vi "Create Message Queue.vi"(8 "error in (no error)":errorcluster, 9 "Initial Message Values":string[](array[string]), 10 "Initial Message Names":string[](array[string]), 11 "Message Queue Name":string) -> (0 "error out":errorcluster, 3 "Message Queue out":T1)   [LabVIEW 2014, in "AMC.lvlib"]
doc: "This VI creates a new local message queue or returns a reference to an existing message queue baseed on the queue name. You can pass in a list of initial messages which will be added to the queue."
uses:
  AMC.lvlib
  _SubVIs/TypeDefs/Message Queue.ctl
  _SubVIs/TypeDefs/Message.ctl
  Keyed Array/KeyedArray.ctl
  Keyed Array/Tools_KeyedArray.lvlib
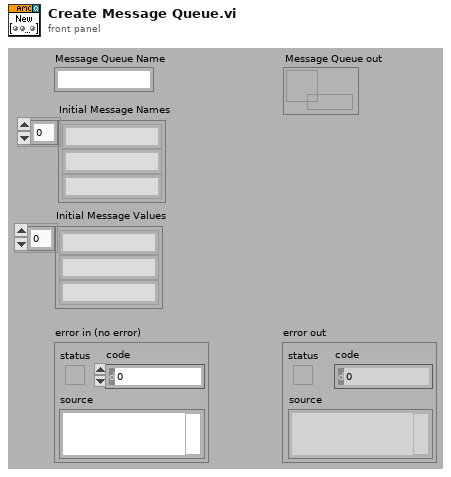
[diagram p1: front panel]
types:
  T1 = typedef "AMC.lvlib/Message Queue.ctl" = refnum<queue>
  T2 = typedef "AMC.lvlib/Message.ctl" = cluster{"Name":string, "Value":string, "Attributes":T3, "Receiver Host":string, "Receiver Process":string, "Source Host":string, "Source Process":string, "Priority Message":bool, "Acknowledge Message":bool}
  T3 = typedef "Tools_KeyedArray.lvlib/KeyedArray.ctl" = cluster{"keys":string[], "values":string[]}
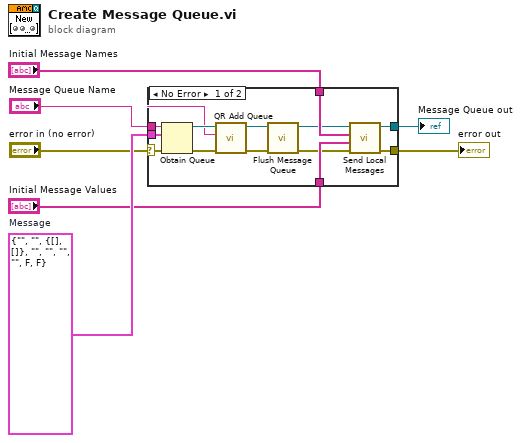
[diagram p0: block diagram]
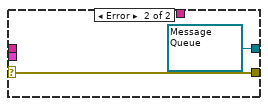
[diagram p2: hidden frame]
diagram:
  w7 = T2 {"Name"="", "Value"="", "Attributes"={"keys"=[], "values"=[]}, "Receiver Host"="", "Receiver Process"="", "Source Host"="", "Source Process"="", "Priority Message"=FALSE, "Acknowledge Message"=FALSE}  # Message
  n1 = case shown="No Error" "error in (no error)" {
    selector: "error in (no error)" -> [w8 w22]
    tunnel: w7 -> [w20 _]
    tunnel: [w19 w22] -> w6
    tunnel: [w18 T1 refnum ("Message Queue out")] -> w5
    tunnel: "Initial Message Names" -> [w17 _]
    tunnel: "Initial Message Values" -> [w16 _]
    tunnel: "Message Queue Name" -> [w13 _]
    frame No Error {
      n2 = Obtain Queue(name (unnamed)=w13, element data type=w20, error in (no error)=w8) -> (queue out=w14:refnum<queue>, error out=w15:errorcluster)  [unwired: 2 in, 1 out]
      n3 = call "QR Add Queue .vi"("error in (no error)"=w15, "Name"=w13, "Message Queue in"=w14) -> ("error out"=w12:errorcluster, "Message Queue out"=w11:T1)  [unwired: 7 out]
      n4 = call "Flush Message Queue.vi"("error in (no error)"=w12, "Message Queue in"=w11) -> ("error out"=w9:errorcluster, "Message Queue out"=w10:T1)  [unwired: 7 out]
      n5 = call "Send Local Messages.vi"("error in (no error)"=w9, "Message Values"=w16, "Message Names"=w17, "Message Queue in"=w10) -> ("error out"=w19:errorcluster, "Message Queue out"=w18:T1)  [unwired: 1 in, 5 out]
    }
    frame Error {
    }
  }
  "Message Queue out" <- w5
  "error out" <- w6
